vi "Test.vi"() -> ()   [LabVIEW 2015]
panel:
  in  "String":string
  out "number (0 to 1)":dbl
  in  "OK Button":bool
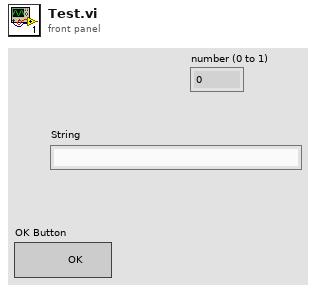
[diagram p1: front panel]
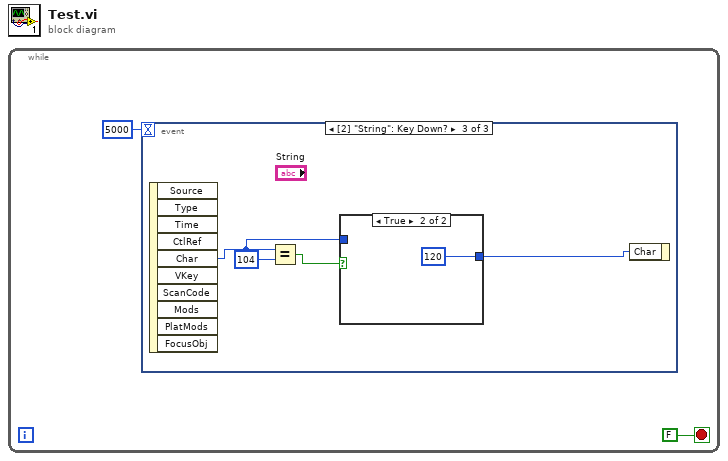
[diagram p0: block diagram]
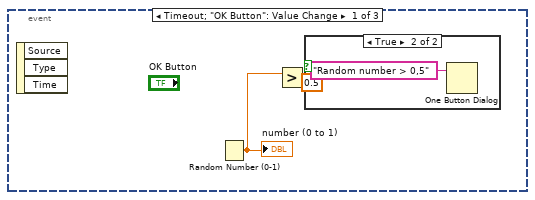
[diagram p2: hidden frame]
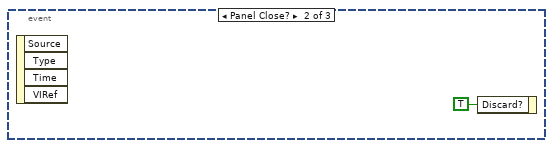
[diagram p4: hidden frame]
diagram:
  n1 = while {
    stop <- FALSE stop-if-true
    n2 = event shown="[2] \"String\": Key Down?" {
      selector: _ -> [_ _ _]
      dyn-events: _ -> [_ _ _]
      timeout: 5000 -> [_ _ _]
      event Timeout; "OK Button": Value Change {
        n3 = event-data() -> ()  [unwired: 1 in, 3 out]
        n4 = Random Number (0-1)() -> (number: 0 to 1=w5:dbl)
        "number (0 to 1)" <- w5
        n5 = Greater?(x=w5, y=0.5) -> (0:w3:bool)
        n6 = case shown="True" w3 {
          frame False {
          }
          frame True {
            n7 = One Button Dialog(message="Random number > 0,5") -> ()  [unwired: 1 in, 1 out]
          }
        }
      }
      event Panel Close? {
        n8 = event-data() -> ()  [unwired: 1 in, 4 out]
        n9 = event-data("Discard?"=TRUE) -> ()  [unwired: 1 in, 1 out]
      }
      event "String": Key Down? {
        n10 = event-data() -> ("Char"=w9:i16)  [unwired: 1 in, 9 out]
        n11 = Equal?(x=w9, y=i16 104) -> (x = y?=w11:bool)
        n12 = case shown="True" w11 {
          tunnel: [w12 i16 120 ("Char")] -> w10
          tunnel: w9 -> [w12 _]
          frame False {
          }
          frame True {
          }
        }
        n13 = event-data("Char"=w10) -> ()  [unwired: 1 in, 1 out]
      }
    }
  }
